vi "Set AutoSize.vi"(8 "error in":errorcluster, 10 "Autosize?":bool, 11 "SourceGrid in":refnum<class "SourceGrid.lvclass">) -> (0 "error out":errorcluster, 3 "SourceGrid out":refnum<class "SourceGrid.lvclass">)   [LabVIEW 2024]
uses:
  SourceGrid.lvclass
  SourceGrid.lvclass/SourceGrid.ctl
  D:/git/Sourcegrid-LabVIEW/dll/SourceGrid.dll
  dll/SourceGrid.dll
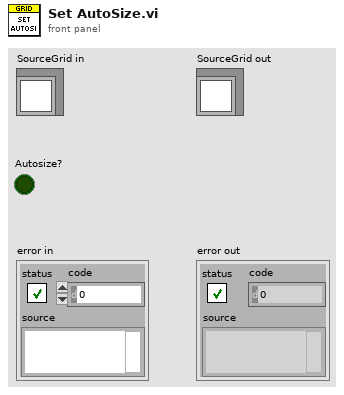
[diagram p1: front panel]
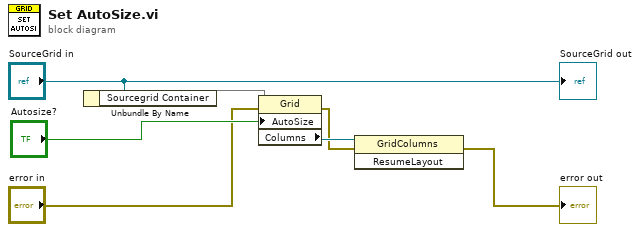
[diagram p0: block diagram]
diagram:
  n1 = Unbundle By Name("SourceGrid in") -> ("Sourcegrid Container"=w6)
  n2 = property class="Grid"(reference=w6, error in="error in", "AutoSize"="Autosize?") -> (error out=w2:errorcluster, "Columns"=w3:refnum<k24>)  [unwired: 1 out]
  n3 = invoke class="GridColumns" method="ResumeLayout"(reference=w3, error in=w2) -> (error out=→"error out":errorcluster)  [unwired: 1 in, 2 out]
  "SourceGrid out" <- "SourceGrid in"
